vi "SS2 Live_Internal Data Storage.vi"(6 "Get(F)/Set":bool, 7 "SS2 Live Data":T3, 8 "Error In":errorcluster, 11 "Variant":variant) -> (0 "Error Out":errorcluster, 1 "Found/Replaced?":bool, 3 "Variant":variant)   [LabVIEW 2019]
uses:
  SS2 Live_Internal Data List.ctl
  SS2 Live_File Saving Task Information.ctl
  73672683-f5cc-4f44-afc7-723f83c649f1.vi
panel:
  in  "Current Image ROI Descriptor":T1 {"Contours"."Type" items=["No Selection", "Point", "Line", "Rectangle", "Oval", "Polygon", "Freehand Region", "Annulus", "Unused2", "Unused3", "Broken Line", "Freehand Line", "Rotated Rectangle"]}
  in  "File Saving Tasks Information":T2[](array[typedef])
  in  "Number of pending file saving tasks":i32
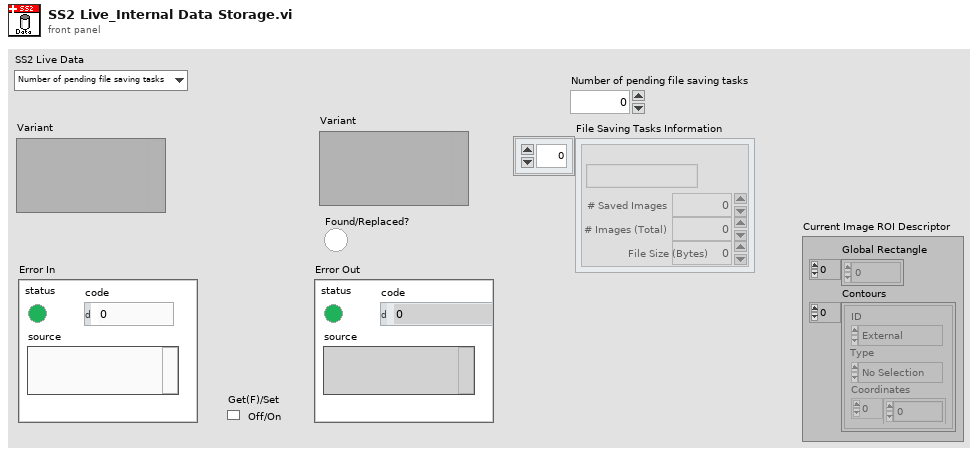
[diagram p1: front panel]
types:
  T1 = typedef "ROI Descriptor" = cluster{"Global Rectangle":i32[], "Contours":cluster{"ID":enum32{"External", "Internal"}, "Type":u32, "Coordinates":i32[]}[]}
  T2 = typedef "SS2 Live_File Saving Task Information.ctl" = cluster{"File Path":string, "# Saved Images":i32, "# Images (Total)":i32, "File Size (Bytes)":i64}
  T3 = typedef "SS2 Live_Internal Data List.ctl" = enum16{"Number of pending file saving tasks", "File Saving Tasks Information", "Current Image ROI Information"}
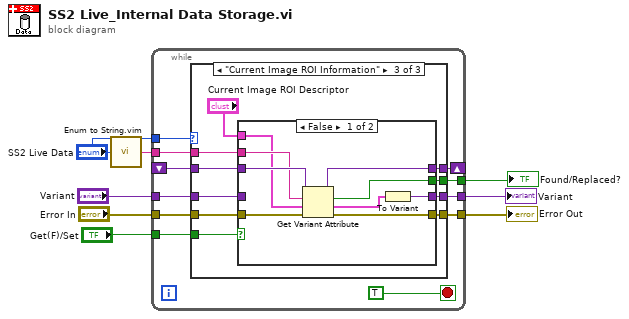
[diagram p0: block diagram]
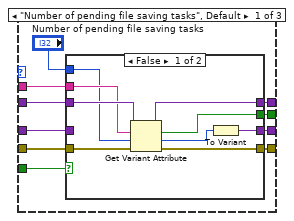
[diagram p2: hidden frame]
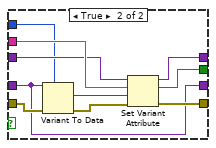
[diagram p3: hidden frame]
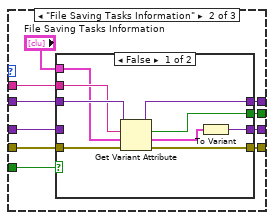
[diagram p4: hidden frame]
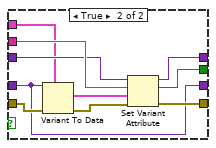
[diagram p5: hidden frame]
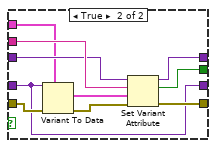
[diagram p6: hidden frame]
diagram:
  n1 = call "Enum to String.vim"("Enum"="SS2 Live Data") -> ("String"=w6:string)
  n2 = while {
    tunnel: "Get(F)/Set" -> [w18]
    shift-right: [w14] -> _
    shift-left: _ -> [w13]
    tunnel: "Variant" -> [w17]
    tunnel: w6 -> [w16]
    tunnel: "Error In" -> [w15]
    tunnel: [w12] -> w4
    tunnel: [w11] -> w3
    tunnel: [w10] -> w2
    tunnel: "SS2 Live Data" -> [w9]
    stop <- TRUE stop-if-true
    n3 = case shown="\"Current Image ROI Information\"" w9 {
      tunnel: w18 -> [w29 w58 w87]
      tunnel: w17 -> [w28 w57 w86]
      tunnel: w16 -> [w27 w56 w85]
      tunnel: w15 -> [w26 w55 w84]
      tunnel: [w25 w54 w83] -> w14
      tunnel: w13 -> [w24 w53 w82]
      tunnel: [w23 w52 w81] -> w12
      tunnel: [w22 w51 w80] -> w11
      tunnel: [w21 w50 w79] -> w10
      frame "Number of pending file saving tasks", Default {
        n4 = case shown="False" w29 {
          tunnel: w28 -> [_ w40]
          tunnel: w27 -> [w36 w48]
          tunnel: w26 -> [w35 w43]
          tunnel: [w37 w47] -> w25
          tunnel: w24 -> [w38 w46]
          tunnel: [w34 w45] -> w23
          tunnel: [w31 w40] -> w22
          tunnel: [w32 w44] -> w21
          tunnel: "Number of pending file saving tasks" -> [w30 w39]
          frame False {
            n5 = Get Variant Attribute(Variant=w38, name=w36, default value (empty Variant)=w30, error in=w35) -> (duplicate Variant=w37:variant, found=w32:bool, value=w33:i32, error out=w34:errorcluster)
            n6 = To Variant(anything=w33) -> (Variant=w31:variant)
          }
          frame True {
            n7 = Variant To Data(error in=w43, type=w39, Variant=w40) -> (data=w41:i32, error out=w42:errorcluster)
            n8 = Set Variant Attribute(Variant=w46, name=w48, value=w41, error in=w42) -> (Variant out=w47:variant, replaced=w44:bool, error out=w45:errorcluster)
          }
        }
      }
      frame "File Saving Tasks Information" {
        n9 = case shown="False" w58 {
          tunnel: w57 -> [_ w69]
          tunnel: w56 -> [w65 w77]
          tunnel: w55 -> [w64 w72]
          tunnel: [w66 w76] -> w54
          tunnel: w53 -> [w67 w75]
          tunnel: [w63 w74] -> w52
          tunnel: [w60 w69] -> w51
          tunnel: [w61 w73] -> w50
          tunnel: "File Saving Tasks Information" -> [w59 w68]
          frame False {
            n10 = Get Variant Attribute(Variant=w67, name=w65, default value (empty Variant)=w59, error in=w64) -> (duplicate Variant=w66:variant, found=w61:bool, value=w62:T2[], error out=w63:errorcluster)
            n11 = To Variant(anything=w62) -> (Variant=w60:variant)
          }
          frame True {
            n12 = Variant To Data(error in=w72, type=w68, Variant=w69) -> (data=w70:T2[], error out=w71:errorcluster)
            n13 = Set Variant Attribute(Variant=w75, name=w77, value=w70, error in=w71) -> (Variant out=w76:variant, replaced=w73:bool, error out=w74:errorcluster)
          }
        }
      }
      frame "Current Image ROI Information" {
        n14 = case shown="False" w87 {
          tunnel: w86 -> [_ w98]
          tunnel: w85 -> [w94 w106]
          tunnel: w84 -> [w93 w101]
          tunnel: [w95 w105] -> w83
          tunnel: w82 -> [w96 w104]
          tunnel: [w92 w103] -> w81
          tunnel: [w89 w98] -> w80
          tunnel: [w90 w102] -> w79
          tunnel: "Current Image ROI Descriptor" -> [w88 w97]
          frame False {
            n15 = Get Variant Attribute(Variant=w96, name=w94, default value (empty Variant)=w88, error in=w93) -> (duplicate Variant=w95:variant, found=w90:bool, value=w91:T1, error out=w92:errorcluster)
            n16 = To Variant(anything=w91) -> (Variant=w89:variant)
          }
          frame True {
            n17 = Variant To Data(error in=w101, type=w97, Variant=w98) -> (data=w99:T1, error out=w100:errorcluster)
            n18 = Set Variant Attribute(Variant=w104, name=w106, value=w99, error in=w100) -> (Variant out=w105:variant, replaced=w102:bool, error out=w103:errorcluster)
          }
        }
      }
    }
  }
  "Error Out" <- w4
  "Variant" <- w3
  "Found/Replaced?" <- w2
